vi "At Line.vi"(10 "Line":T1, 11 "Brick Wall in":refnum<class "Brick Wall.lvclass">) -> (3 "At Line":bool)   [LabVIEW 2015, in "Brick Wall.lvclass"]
uses:
  Brick Wall.lvclass
  Type Defs/Direction Enum.ctl
  Brick Wall.lvclass/Brick Wall.ctl
  Type Defs/SB Type Defs.lvlib
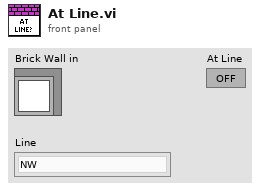
[diagram p1: front panel]
types:
  T1 = typedef "SB Type Defs.lvlib/Direction Enum.ctl" = enum16{"NW", "N", "NE", "E", "SE", "S", "SW", "W"}
  T2 = typedef "Brick Wall.lvclass/MasonLines.ctl" = cluster{"NMasonLine":i32, "EMasonLine":i32, "SMasonLine":i32, "WMasonLine":i32}
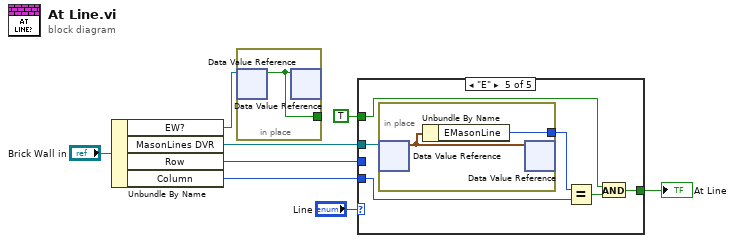
[diagram p0: block diagram]
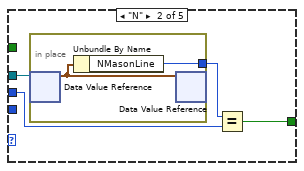
[diagram p3: hidden frame]
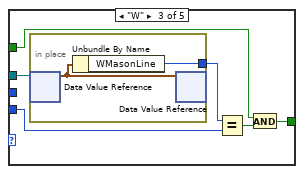
[diagram p4: hidden frame]
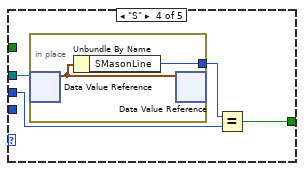
[diagram p5: hidden frame]
diagram:
  n1 = Unbundle By Name("Brick Wall in") -> ("EW?"=w2:refnum<data-value>, "MasonLines DVR"=w5:refnum<data-value>, "Row"=w6:i32, "Column"=w3:i32)
  n2 = in-place {
    in-place-border: [w9] -> _
    n3 = in-place-dvr #1(w2) -> (w9:bool)  [unwired: 1 out]
    n4 = in-place-dvr #1(w9) -> ()  [unwired: 2 out]
  }
  n5 = case shown="\"E\"" "Line" {
    tunnel: w5 -> [_ w13 w21 w27 w35]
    tunnel: w6 -> [_ w11 _ w25 _]
    tunnel: [_ w10 w17 w24 w31] -> w7
    tunnel: w3 -> [_ _ w18 _ w32]
    tunnel: TRUE -> [_ _ w16 _ w30]
    frame Default {
    }
    frame "N" {
      n6 = in-place {
        in-place-border: [w14] -> w12
        n7 = in-place-dvr #2(w13) -> (w15:T2)  [unwired: 1 out]
        n8 = Unbundle By Name(w15) -> ("NMasonLine"=w14:i32)
        n9 = in-place-dvr #2(w15) -> ()  [unwired: 2 out]
      }
      n10 = Equal?(x=w12, y=w11) -> (x = y?=w10:bool)
    }
    frame "W" {
      n11 = in-place {
        in-place-border: [w22] -> w20
        n12 = in-place-dvr #3(w21) -> (w23:T2)  [unwired: 1 out]
        n13 = Unbundle By Name(w23) -> ("WMasonLine"=w22:i32)
        n14 = in-place-dvr #3(w23) -> ()  [unwired: 2 out]
      }
      n15 = Equal?(x=w20, y=w18) -> (x = y?=w19:bool)
      n16 = And(x=w16, y=w19) -> (x .and. y?=w17:bool)
    }
    frame "S" {
      n17 = in-place {
        in-place-border: [w28] -> w26
        n18 = in-place-dvr #4(w27) -> (w29:T2)  [unwired: 1 out]
        n19 = Unbundle By Name(w29) -> ("SMasonLine"=w28:i32)
        n20 = in-place-dvr #4(w29) -> ()  [unwired: 2 out]
      }
      n21 = Equal?(x=w26, y=w25) -> (x = y?=w24:bool)
    }
    frame "E" {
      n22 = in-place {
        in-place-border: [w36] -> w34
        n23 = in-place-dvr #5(w35) -> (w37:T2)  [unwired: 1 out]
        n24 = Unbundle By Name(w37) -> ("EMasonLine"=w36:i32)
        n25 = in-place-dvr #5(w37) -> ()  [unwired: 2 out]
      }
      n26 = Equal?(x=w34, y=w32) -> (x = y?=w33:bool)
      n27 = And(x=w30, y=w33) -> (x .and. y?=w31:bool)
    }
  }
  "At Line" <- w7
